vi "Do.vi"(8 "error in (no error)":errorcluster, 10 "Actor in":refnum<class "Actor.lvclass">, 11 "Integral Msg":refnum<class "Integral Msg.lvclass">) -> (0 "error out":errorcluster, 2 "Actor out":refnum<class "Actor.lvclass">)   [LabVIEW 2015, in "KIT-QA.lvlib" / "Integral Msg.lvclass"]
doc: "This VI delivers the message to the actor by calling the appropriate method(s) on the actor."
uses:
  Integral Msg.lvclass
  <vilib>/ActorFramework/Actor/Actor.lvclass
  KIT-QA/KIT-QA.lvclass
  Integral Msg.lvclass/Integral Msg.ctl
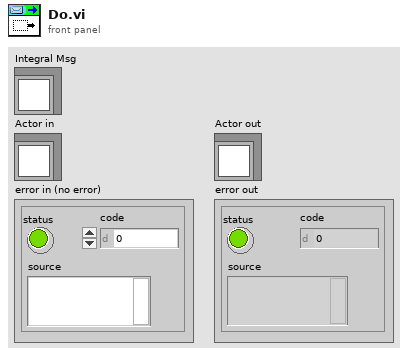
[diagram p1: front panel]
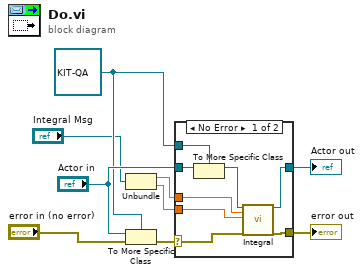
[diagram p0: block diagram]
diagram:
  w4 = refnum<class "KIT-QA.lvclass"> refnum ("Actor in")
  n1 = Unbundle ("Main-Unbundle")("Integral Msg") -> (w2:dbl, w1:dbl)
  n2 = To More Specific Class(target class=w4, reference="Actor in", error in="error in (no error)") -> (error out=w8:errorcluster)  [unwired: 1 out]
  n3 = case shown="No Error" w8 {
    selector: w8 -> [w15 w19]
    tunnel: [w17 w19] -> w7
    tunnel: [w16 w18] -> w6
    tunnel: "Actor in" -> [w14 w18]
    tunnel: w4 -> [w13 _]
    tunnel: w2 -> [w11 _]
    tunnel: w1 -> [w10 _]
    frame No Error {
      n4 = To More Specific Class(target class=w13, reference=w14) -> (specific class reference=w12:refnum<class "KIT-QA.lvclass">)  [unwired: 1 in, 1 out]
      n5 = call "Integral.vi"("KIT-QA in"=w12, "-t1"=w11, "t100"=w10, "error in (no error)"=w15) -> ("KIT-QA out"=w16:refnum<class "KIT-QA.lvclass">, "error out"=w17:errorcluster)  [unwired: 12 in, 2 out]
    }
    frame Error {
    }
  }
  "error out" <- w7
  "Actor out" <- w6
